vi "Coordinate_Outlier_Filtering_R1.vi"(0 "Num of Beacons":i8=5, 1 "Max Std Dev(all 5)":dbl=1.0, 5 "X in":sgl[](array[numeric]), 7 "Valid Data\nSets in":bool[](array[boolean])=[TRUE, TRUE, TRUE, TRUE, TRUE], 9 "Y in":sgl[](array[numeric]), 11 "Max Std Dev( 4 )":dbl=1.0, 13 "Max Std Dev (3)":dbl=1.0) -> (3 "Y out":sgl[](array[numeric]), 4 "Max":i32, 6 "Min Std Dev\nfor Max beacons":dbl, 8 "X out":sgl[](array[numeric]), 10 "Valid Beacons\nout":bool[](array[boolean]), 15 "Slope out":dbl)   [LabVIEW 2015]
uses:
  <vilib>/Analysis/NI_AALPro.lvlib
panel:
  out "std dev_current":dbl format="%0.6f"
  out "std dev_current 3":dbl format="%0.6f"
  out "size(s) 2":i32
  out "std dev_current 2":dbl format="%0.6f"
  out "size(s)":i32
  in  "Combo_info\nTemplate":T1={"Num Beacons"=0, "Std Dev_combo"=0.0, "Valid Data\nSets_combo"=[FALSE, FALSE, FALSE, FALSE, FALSE], "Slope combo"=0.0}
types:
  T1 = cluster{"Num Beacons":u8, "Std Dev_combo":dbl, "Valid Data\nSets_combo":bool[], "Slope combo":dbl}
  T2 = cluster{"dimension size":u8, sgl, bool[], "slope":dbl}
  T3 = cluster{"dimension size":u8, "Std Dev_combo":dbl, "Valid Data\nSets_combo":bool[], "slope":dbl}[]
  T4 = cluster{"dimension size":u8, dbl, bool[], "slope":dbl}
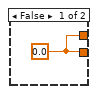
[diagram p2: hidden frame]
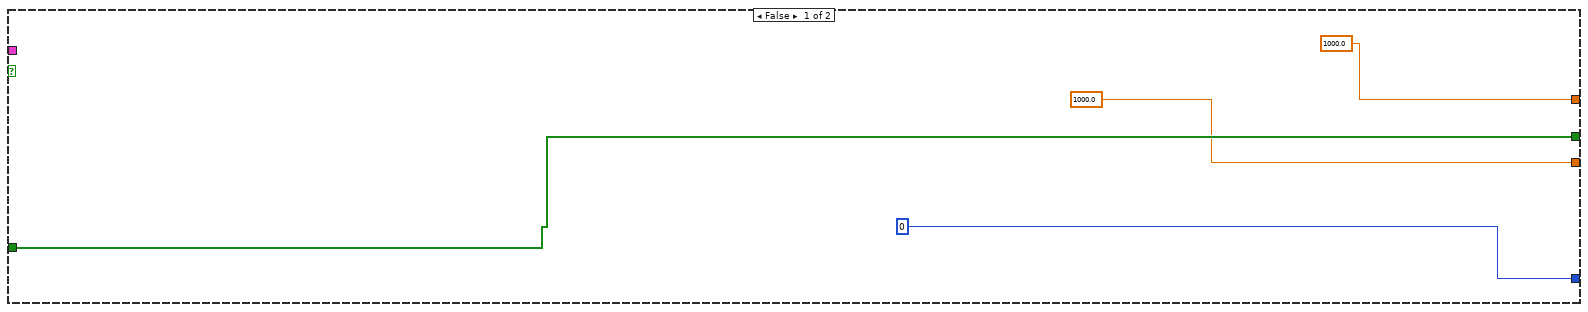
[diagram p3: hidden frame]
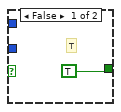
[diagram p8: hidden frame]
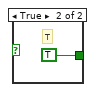
[diagram p9: hidden frame]
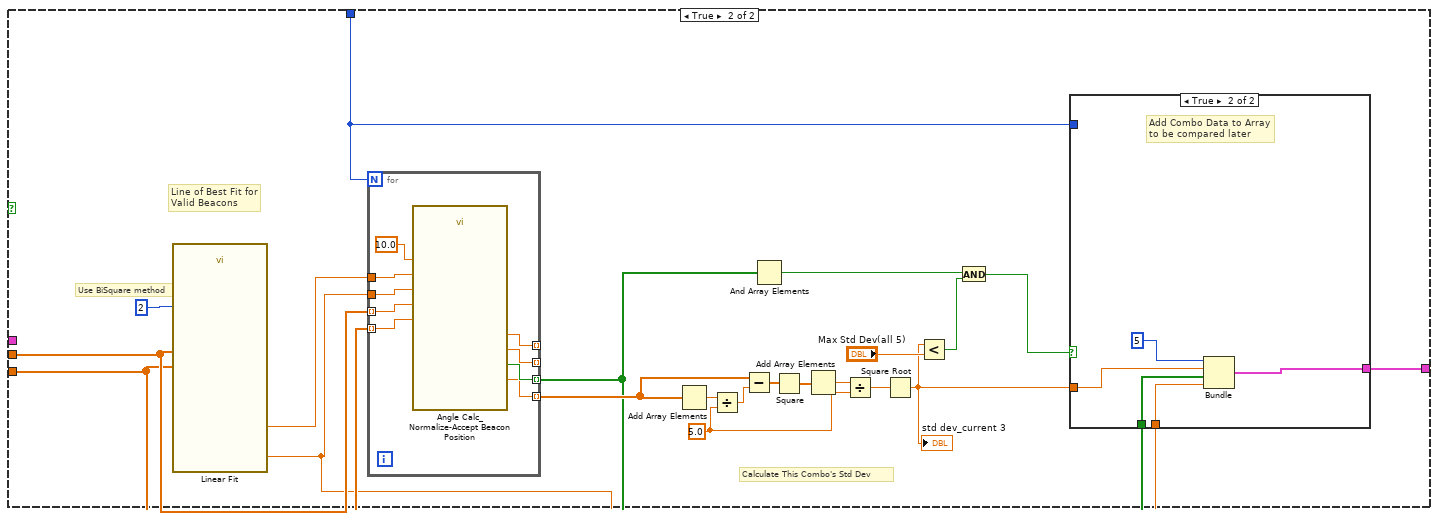
[diagram p13: hidden frame]
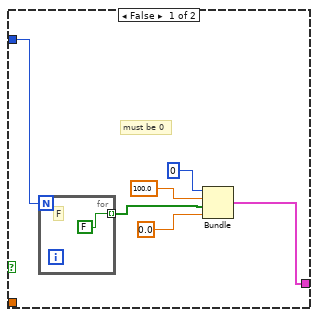
[diagram p14: hidden frame]
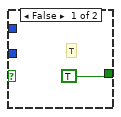
[diagram p16: hidden frame]
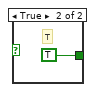
[diagram p17: hidden frame]
diagram:
  # "Use BiSquare method"
  # "Line of Best Fit for\nValid Beacons"
  # "5  Beacon Combination (only 1)"
  # "4 Beacon Combinations"
  # "3 Beacon Combinations"
  n1 = Boolean To (0,1)(Boolean="Valid Data\nSets in") -> (0, 1=w39:i16[])
  n2 = Add Array Elements(numeric array=w39) -> (sum=w26:i16)
  n3 = Equal?(x=w26, y=5 ("dimension size")) -> (x = y?=w34:bool)
  n4 = case shown="False" w34 {
    tunnel: "X in" -> [_ w59]
    tunnel: "Y in" -> [_ w58]
    tunnel: "Num of Beacons" -> [_ w43]
    tunnel: [w40 w44] -> w32
    tunnel: "Combo_info\nTemplate" -> [w40 _]
    frame False {
    }
    frame True {
      w42 = sgl 5.0 ("y")
      # "Calculate This Combo's Std Dev"
      # "Use BiSquare method"
      # "Line of Best Fit for\nValid Beacons"
      n5 = call <vilib>:"Linear Fit.vi"("Y"=w58, "X"=w59, "method"=2) -> ("slope"=w41:dbl, "intercept"=w60:dbl)  [unwired: 8 in, 3 out]
      n6 = for {
        N: w43 -> [_]
        tunnel: w41 -> [w81]
        tunnel: w60 -> [w80]
        tunnel: w59 -> [w79] mode=indexing
        tunnel: w58 -> [w78] mode=indexing
        tunnel: [w77] -> w45 mode=indexing
        tunnel: [w76] -> w46 mode=indexing
        tunnel: [w75] -> _ mode=indexing
        tunnel: [w74] -> _ mode=indexing
        n7 = call "Angle Calc_Normalize-Accept Beacon Position.vi"("slope"=w81, "Xin"=w79, "Deviation Threshold"=sgl 10.0 ("Deviation Threshold\n- Local Beacon Pos(*unit)"), "intercept"=w80, "Yin"=w78) -> ("Accept Beacon"=w77:bool, "Xout"=w75:sgl, "Distance"=w76:sgl, "Yout"=w74:sgl)  [unwired: 6 in, 1 out]
      }
      n8 = Add Array Elements(numeric array=w46) -> (sum=w57:sgl)
      n9 = Divide(x=w57, y=w42) -> (x/y=w56:sgl)
      n10 = Subtract(x=w46, y=w56) -> (x-y=w55:sgl[])
      n11 = And Array Elements(Boolean array=w45) -> (logical AND=w51:bool)
      n12 = Square(x=w55) -> (x^2=w47:sgl[])
      n13 = Add Array Elements(numeric array=w47) -> (sum=w53:sgl)
      n14 = Divide(x=w53, y=w42) -> (x/y=w54:sgl)
      n15 = Square Root(x=w54) -> (sqrt(x)=w49:sgl)
      "std dev_current 3" <- w49
      n16 = Less?(x=w49, y="Max Std Dev(all 5)") -> (x < y?=w50:bool)
      n17 = And(x=w51, y=w50) -> (x .and. y?=w48:bool)
      n18 = case shown="True" w48 {
        tunnel: w49 -> [_ w72]
        tunnel: w45 -> [_ w71]
        tunnel: [w64 w70] -> w44
        tunnel: w43 -> [w63 _]
        tunnel: w41 -> [_ w69]
        frame False {
          # "must be 0"
          n19 = for {
            N: w63 -> [_]
            tunnel: [FALSE] -> w65 mode=indexing
            # "F"
          }
          n20 = Bundle("dimension size"=u8 0, 100.0, w65, 0.0) -> (w64:cluster{"dimension size":u8, dbl, bool[], dbl})  [unwired: 1 in]
        }
        frame True {
          # "Add Combo Data to Array\nto be compared later"
          n21 = Bundle("dimension size"=u8 5, w72, w71, "slope"=w69) -> (w70:T2)  [unwired: 1 in]
        }
      }
    }
  }
  n22 = Build Array(w32) -> (w30:T3)
  n23 = Greater Or Equal?(x=w26, y=i16 4) -> (x >= y?=w37:bool)
  n24 = case shown="True" w37 {
    tunnel: "Num of Beacons" -> [_ w87]
    tunnel: "X in" -> [_ w90]
    tunnel: "Y in" -> [_ w89]
    tunnel: "Valid Data\nSets in" -> [_ w88]
    tunnel: w30 -> [w83 w86]
    tunnel: [w83 w85] -> w29
    tunnel: "Num of Beacons" -> [_ w84]
    frame False {
    }
    frame True {
      n25 = for {
        N: w87 -> [w94]
        shift-right: [w92] -> w85
        shift-left: w86 -> [w93]
        tunnel: w90 -> [w97]
        tunnel: w89 -> [w96]
        tunnel: w88 -> [w98]
        tunnel: w84 -> [w91]
        i -> [w95]
        n26 = for {
          N: w94 -> [w102]
          tunnel: w95 -> [w104]
          shift-right: [w100] -> w92
          shift-left: w93 -> [w101]
          tunnel: w97 -> [w106]
          tunnel: w96 -> [w105]
          tunnel: w98 -> [w107]
          tunnel: w91 -> [w99]
          i -> [w103]
          n27 = for {
            N: w102 -> [w110]
            tunnel: w107 -> [w116]
            tunnel: w106 -> [w115]
            tunnel: w105 -> [w114]
            tunnel: w104 -> [w111]
            tunnel: w103 -> [w117]
            shift-right: [w113] -> w100
            shift-left: w101 -> [w109]
            tunnel: w99 -> [w108]
            i -> [w112]
            n28 = for {
              N: w110 -> [w127]
              tunnel: w117 -> [w129]
              tunnel: w116 -> [w152]
              tunnel: w115 -> [w150]
              tunnel: w114 -> [w149]
              tunnel: w112 -> [w130]
              tunnel: w111 -> [w128]
              shift-right: [w139] -> w113
              shift-left: w109 -> [w131]
              tunnel: w108 -> [w118]
              i -> [w126]
              w132 = 4
              # "Build Beacon Set Boolean Array\n(correlates to indexes)"
              # "Fetch Coordinates"
              # "Are All Indexes Different?\nAND\nDo those indexes contain valid beacons?\nAND\nIs it not a repeat combo?"
              n29 = Greater?(x=w130, y=w129) -> (0:w122:bool)
              n30 = Greater?(x=w129, y=w128) -> (0:w123:bool)
              n31 = Greater?(x=w126, y=w130) -> (0:w121:bool)
              n32 = Build Array(w128, w129, w130, w126) -> (w137:i32[])
              n33 = for {
                N: w132 -> [_]
                tunnel: w137 -> [w156] mode=indexing
                tunnel: w137 -> [w157]
                tunnel: [w154] -> w136 mode=indexing
                tunnel: w132 -> [w153]
                i -> [w158]
                n34 = for {
                  N: w153 -> [_]
                  tunnel: w158 -> [w163]
                  tunnel: w157 -> [w161] mode=indexing
                  tunnel: w156 -> [w160]
                  tunnel: [w159] -> w155 mode=indexing
                  i -> [w162]
                  n35 = Not Equal?(x=w163, y=w162) -> (x != y?=w164:bool)
                  n36 = case shown="True" w164 {
                    tunnel: w161 -> [_ w167]
                    tunnel: w160 -> [_ w166]
                    tunnel: [TRUE w168] -> w159
                    frame False {
                      # "T"
                    }
                    frame True {
                      n37 = Not Equal?(x=w166, y=w167) -> (x != y?=w168:bool)
                    }
                  }
                }
                n38 = And Array Elements(Boolean array=w155) -> (logical AND=w154:bool)
              }
              n39 = And Array Elements(Boolean array=w136) -> (logical AND=w120:bool)
              n40 = Index Array(array=w150, index #1=w128, index #2=w129, index #3=w130, index #4=w126) -> (element #1=w148:sgl, element #2=w147:sgl, element #3=w146:sgl, element #4=w125:sgl)
              n41 = Index Array(array=w149, index #1=w128, index #2=w129, index #3=w130, index #4=w126) -> (element #1=w145:sgl, element #2=w144:sgl, element #3=w143:sgl, element #4=w124:sgl)
              n42 = Index Array(array=w152, index #1=w128, index #2=w129, index #3=w130, index #4=w126) -> (element #1=w135:bool, element #2=w134:bool, element #3=w133:bool, element #4=w119:bool)
              n43 = for {
                N: w127 -> [_]
                tunnel: w130 -> [w179]
                tunnel: w129 -> [w178]
                tunnel: w128 -> [w177]
                tunnel: [w172] -> w138 mode=indexing
                tunnel: w126 -> [w170]
                i -> [w171]
                n44 = Equal?(x=w177, y=w171) -> (x = y?=w174:bool)
                n45 = Equal?(x=w179, y=w171) -> (x = y?=w176:bool)
                n46 = Equal?(x=w178, y=w171) -> (x = y?=w175:bool)
                n47 = Equal?(x=w170, y=w171) -> (x = y?=w169:bool)
                n48 = Compound Arithmetic op=OR(w176, w175, w174, w169) -> (w173:bool)
                n49 = case shown="False" w173 {
                  tunnel: [FALSE TRUE] -> w172
                  frame False {
                    # "F"
                  }
                  frame True {
                    # "T"
                  }
                }
              }
              n50 = Build Array(w148, w147, w146, w125) -> (w142:sgl[])
              n51 = Build Array(w145, w144, w143, w124) -> (w141:sgl[])
              n52 = Build Array(w135, w134, w133, w119) -> (w140:bool[])
              n53 = Compound Arithmetic op=AND(w135, w134, w133, w119, w120, w121, w122, w123) -> (w151:bool)
              n54 = case shown="True" w151 {
                tunnel: w142 -> [_ w200]
                tunnel: w141 -> [_ w201]
                tunnel: w140 -> [_ w191]
                tunnel: w131 -> [w182 w189]
                tunnel: [w182 w187] -> w139
                tunnel: w138 -> [_ w185]
                tunnel: w118 -> [_ w184]
                frame False {
                }
                frame True {
                  # "Calculate Distance from\nBeacon to Fitted Line"
                  # "Calculate This Combo's Std Dev"
                  # "Trim Arrays to Only Valid Beacons"
                  # "Use BiSquare method"
                  # "Line of Best Fit for\nValid Beacons"
                  # "All Indexes are Different and Beacons are Valid"
                  n55 = Initialize Array(sgl 0.0 ("element"), 4 ("dimension size")) -> (w209:sgl[])
                  n56 = for {
                    N: w184 -> [_]
                    shift-right: [w228] -> w198
                    shift-left: 0.0 -> [w229]
                    shift-right: [w227] -> w203
                    shift-left: w209 -> [w226]
                    shift-right: [w224] -> w202
                    shift-left: w209 -> [w225]
                    tunnel: w191 -> [w223] mode=indexing
                    tunnel: w200 -> [w222] mode=indexing
                    tunnel: w201 -> [w221] mode=indexing
                    n57 = case shown="True" w223 {
                      tunnel: w229 -> [w232 w239]
                      tunnel: [w232 w240] -> w228
                      tunnel: [w231 w237] -> w227
                      tunnel: w226 -> [w231 w236]
                      tunnel: w225 -> [w230 w235]
                      tunnel: [w230 w238] -> w224
                      tunnel: w222 -> [_ w234]
                      tunnel: w221 -> [_ w233]
                      frame False {
                      }
                      frame True {
                        n58 = Replace Array Subset(array=w236, new element=w234, index=w239) -> (w237:sgl[])
                        n59 = Replace Array Subset(array=w235, new element=w233, index=w239) -> (w238:sgl[])
                        n60 = Increment(x=w239) -> (x+1=w240:dbl)
                      }
                    }
                  }
                  n61 = call <vilib>:"Linear Fit.vi"("Y"=w202, "X"=w203, "method"=2) -> ("slope"=w183:dbl, "intercept"=w211:dbl)  [unwired: 8 in, 3 out]
                  n62 = for {
                    N: w184 -> [_]
                    tunnel: w211 -> [w249]
                    tunnel: w183 -> [w248]
                    tunnel: w203 -> [w247] mode=indexing
                    tunnel: w202 -> [w246] mode=indexing
                    tunnel: [w245] -> w194 mode=indexing
                    tunnel: [w244] -> _ mode=indexing
                    tunnel: [w243] -> _ mode=indexing
                    tunnel: [w242] -> w196 mode=indexing
                    n63 = call "Angle Calc_Normalize-Accept Beacon Position.vi"("slope"=w248, "Xin"=w247, "Deviation Threshold"=sgl 10.0 ("Deviation Threshold\n- Local Beacon Pos(*unit)"), "intercept"=w249, "Yin"=w246) -> ("Accept Beacon"=w245:bool, "Xout"=w244:sgl, "Distance"=w242:sgl, "Yout"=w243:sgl)  [unwired: 6 in, 1 out]
                  }
                  n64 = Add Array Elements(numeric array=w196) -> (sum=w208:sgl)
                  n65 = Divide(x=w208, y=w198) -> (x/y=w207:dbl)
                  n66 = Subtract(x=w196, y=w207) -> (x-y=w206:dbl[])
                  n67 = And Array Elements(Boolean array=w194) -> (logical AND=w193:bool)
                  n68 = Square(x=w206) -> (x^2=w195:dbl[])
                  n69 = Add Array Elements(numeric array=w195) -> (sum=w204:dbl)
                  n70 = Divide(x=w204, y=w198) -> (x/y=w205:dbl)
                  n71 = Square Root(x=w205) -> (sqrt(x)=w190:dbl)
                  "std dev_current 2" <- w190
                  n72 = Less?(x=w190, y="Max Std Dev( 4 )") -> (x < y?=w192:bool)
                  n73 = And(x=w193, y=w192) -> (x .and. y?=w188:bool)
                  n74 = case shown="True" w188 {
                    tunnel: w185 -> [_ w220]
                    tunnel: w190 -> [_ w219]
                    tunnel: w189 -> [w213 w218]
                    tunnel: [w213 w217] -> w187
                    tunnel: w183 -> [_ w214]
                    frame False {
                    }
                    frame True {
                      # "Add Combo Data to Array\nto be compared later"
                      n75 = Bundle("dimension size"=u8 4, w219, w220, "slope"=w214) -> (w215:T4)  [unwired: 1 in]
                      n76 = Build Array (concatenate)(w218, w215) -> (w217:T3)
                    }
                  }
                }
              }
            }
          }
        }
      }
    }
  }
  n77 = Array Size(array=w29) -> (size(s)=w35:i32)
  n78 = Decrement(x=w35) -> (x-1=w24:i32)
  "size(s) 2" <- w24
  n79 = Greater Or Equal?(x=w26, y=3 ("dimension size")) -> (x >= y?=w27:bool)
  n80 = case shown="True" w27 {
    tunnel: "Num of Beacons" -> [_ w251]
    tunnel: "X in" -> [_ w256]
    tunnel: "Y in" -> [_ w255]
    tunnel: "Valid Data\nSets in" -> [_ w254]
    tunnel: w29 -> [w250 w253]
    tunnel: [w250 w252] -> w21
    frame False {
    }
    frame True {
      n81 = for {
        N: w251 -> [w259]
        shift-right: [w257] -> w252
        shift-left: w253 -> [w258]
        tunnel: w256 -> [w262]
        tunnel: w255 -> [w261]
        tunnel: w254 -> [w263]
        i -> [w260]
        n82 = for {
          N: w259 -> [w266]
          tunnel: w260 -> [w268]
          shift-right: [w264] -> w257
          shift-left: w258 -> [w265]
          tunnel: w262 -> [w270]
          tunnel: w261 -> [w269]
          tunnel: w263 -> [w271]
          i -> [w267]
          n83 = for {
            N: w266 -> [w282]
            tunnel: w271 -> [w300]
            tunnel: w270 -> [w298]
            tunnel: w269 -> [w297]
            tunnel: w268 -> [w272]
            tunnel: w267 -> [w273]
            shift-right: [w283] -> w264
            shift-left: w265 -> [w284]
            i -> [w274]
            w279 = 3
            # "Build Beacon Set Boolean Array\n(correlates to indexes)"
            # "Fetch Coordinates"
            # "Are All Indexes Different?\nAND\nDo those indexes contain valid beacons?\nAND\nIs it not a repeat combo?"
            n84 = Greater?(x=w274, y=w273) -> (0:w276:bool)
            n85 = Greater?(x=w273, y=w272) -> (0:w275:bool)
            n86 = Build Array(w272, w273, w274) -> (w280:i32[])
            n87 = for {
              N: w279 -> [_]
              tunnel: w280 -> [w304] mode=indexing
              tunnel: w280 -> [w305]
              tunnel: [w302] -> w278 mode=indexing
              tunnel: w279 -> [w301]
              i -> [w306]
              n88 = for {
                N: w301 -> [_]
                tunnel: w306 -> [w311]
                tunnel: w305 -> [w309] mode=indexing
                tunnel: w304 -> [w308]
                tunnel: [w307] -> w303 mode=indexing
                i -> [w310]
                n89 = Not Equal?(x=w311, y=w310) -> (x != y?=w312:bool)
                n90 = case shown="True" w312 {
                  tunnel: w309 -> [_ w315]
                  tunnel: w308 -> [_ w314]
                  tunnel: [TRUE w316] -> w307
                  frame False {
                    # "T"
                  }
                  frame True {
                    n91 = Not Equal?(x=w314, y=w315) -> (x != y?=w316:bool)
                  }
                }
              }
              n92 = And Array Elements(Boolean array=w303) -> (logical AND=w302:bool)
            }
            n93 = And Array Elements(Boolean array=w278) -> (logical AND=w277:bool)
            n94 = Index Array(array=w298, index #1=w272, index #2=w273, index #3=w274) -> (element #1=w296:sgl, element #2=w295:sgl, element #3=w294:sgl)
            n95 = Index Array(array=w297, index #1=w272, index #2=w273, index #3=w274) -> (element #1=w293:sgl, element #2=w292:sgl, element #3=w291:sgl)
            n96 = for {
              N: w282 -> [_]
              tunnel: w274 -> [w324]
              tunnel: w273 -> [w323]
              tunnel: w272 -> [w322]
              tunnel: [w317] -> w281 mode=indexing
              i -> [w325]
              n97 = Equal?(x=w322, y=w325) -> (x = y?=w319:bool)
              n98 = Equal?(x=w324, y=w325) -> (x = y?=w321:bool)
              n99 = Equal?(x=w323, y=w325) -> (x = y?=w320:bool)
              n100 = Compound Arithmetic op=OR(w321, w320, w319) -> (w318:bool)
              n101 = case shown="False" w318 {
                tunnel: [FALSE TRUE] -> w317
                frame False {
                  # "F"
                }
                frame True {
                  # "T"
                }
              }
            }
            n102 = Index Array(array=w300, index #1=w272, index #2=w273, index #3=w274) -> (element #1=w288:bool, element #2=w290:bool, element #3=w289:bool)
            n103 = Build Array(w296, w295, w294) -> (w287:sgl[])
            n104 = Build Array(w293, w292, w291) -> (w286:sgl[])
            n105 = Build Array(w288, w290, w289) -> (w285:bool[])
            n106 = Compound Arithmetic op=AND(w288, w290, w289, w277, w276, w275) -> (w299:bool)
            n107 = case shown="True" w299 {
              tunnel: w287 -> [_ w346]
              tunnel: w286 -> [_ w347]
              tunnel: w285 -> [_ w337]
              tunnel: w282 -> [_ w332]
              tunnel: w284 -> [w328 w335]
              tunnel: [w328 w333] -> w283
              tunnel: w281 -> [_ w330]
              frame False {
              }
              frame True {
                # "Calculate Distance from\nBeacon to Fitted Line"
                # "Calculate This Combo's Std Dev"
                # "Trim Arrays to Only Valid Beacons"
                # "Use BiSquare method"
                # "Line of Best Fit for\nValid Beacons"
                # "All Indexes are Different and Beacons are Valid"
                n108 = Initialize Array(sgl 0.0 ("element"), 3 ("dimension size")) -> (w355:sgl[])
                n109 = for {
                  N: w332 -> [_]
                  shift-right: [w374] -> w344
                  shift-left: 0.0 -> [w375]
                  shift-right: [w373] -> w349
                  shift-left: w355 -> [w372]
                  shift-right: [w370] -> w348
                  shift-left: w355 -> [w371]
                  tunnel: w337 -> [w369] mode=indexing
                  tunnel: w346 -> [w368] mode=indexing
                  tunnel: w347 -> [w367] mode=indexing
                  n110 = case shown="True" w369 {
                    tunnel: w375 -> [w378 w385]
                    tunnel: [w378 w386] -> w374
                    tunnel: [w377 w383] -> w373
                    tunnel: w372 -> [w377 w382]
                    tunnel: w371 -> [w376 w381]
                    tunnel: [w376 w384] -> w370
                    tunnel: w368 -> [_ w380]
                    tunnel: w367 -> [_ w379]
                    frame False {
                    }
                    frame True {
                      n111 = Replace Array Subset(array=w382, new element=w380, index=w385) -> (w383:sgl[])
                      n112 = Replace Array Subset(array=w381, new element=w379, index=w385) -> (w384:sgl[])
                      n113 = Increment(x=w385) -> (x+1=w386:dbl)
                    }
                  }
                }
                n114 = call <vilib>:"Linear Fit.vi"("Y"=w348, "X"=w349, "method"=2) -> ("slope"=w329:dbl, "intercept"=w357:dbl)  [unwired: 8 in, 3 out]
                n115 = for {
                  N: w332 -> [_]
                  tunnel: w357 -> [w395]
                  tunnel: w329 -> [w394]
                  tunnel: w349 -> [w393] mode=indexing
                  tunnel: w348 -> [w392] mode=indexing
                  tunnel: [w391] -> w340 mode=indexing
                  tunnel: [w390] -> _ mode=indexing
                  tunnel: [w389] -> _ mode=indexing
                  tunnel: [w388] -> w342 mode=indexing
                  n116 = call "Angle Calc_Normalize-Accept Beacon Position.vi"("slope"=w394, "Xin"=w393, "Deviation Threshold"=sgl 10.0 ("Deviation Threshold\n- Local Beacon Pos(*unit)"), "intercept"=w395, "Yin"=w392) -> ("Accept Beacon"=w391:bool, "Xout"=w390:sgl, "Distance"=w388:sgl, "Yout"=w389:sgl)  [unwired: 6 in, 1 out]
                }
                n117 = Add Array Elements(numeric array=w342) -> (sum=w354:sgl)
                n118 = Divide(x=w354, y=w344) -> (x/y=w353:dbl)
                n119 = Subtract(x=w342, y=w353) -> (x-y=w352:dbl[])
                n120 = And Array Elements(Boolean array=w340) -> (logical AND=w339:bool)
                n121 = Square(x=w352) -> (x^2=w341:dbl[])
                n122 = Add Array Elements(numeric array=w341) -> (sum=w350:dbl)
                n123 = Divide(x=w350, y=w344) -> (x/y=w351:dbl)
                n124 = Square Root(x=w351) -> (sqrt(x)=w336:dbl)
                "std dev_current" <- w336
                n125 = Less?(x=w336, y="Max Std Dev (3)") -> (x < y?=w338:bool)
                n126 = And(x=w339, y=w338) -> (x .and. y?=w334:bool)
                n127 = case shown="True" w334 {
                  tunnel: w330 -> [_ w366]
                  tunnel: w336 -> [_ w365]
                  tunnel: w335 -> [w359 w364]
                  tunnel: [w359 w363] -> w333
                  tunnel: w329 -> [_ w360]
                  frame False {
                  }
                  frame True {
                    # "Add Combo Data to Array\nto be compared later"
                    n128 = Bundle("dimension size"=u8 3, w365, w366, "slope"=w360) -> (w361:T4)  [unwired: 1 in]
                    n129 = Build Array (concatenate)(w364, w361) -> (w363:T3)
                  }
                }
              }
            }
          }
        }
      }
    }
  }
  n130 = Array Size(array=w21) -> (size(s)=w2:i32)
  n131 = Initialize Array(FALSE, 5 ("dimension size")) -> (w15:bool[])
  n132 = Greater Than 0?(x=w2) -> (x > 0?=w20:bool)
  n133 = case shown="True" w20 {
    tunnel: w2 -> [_ w407]
    tunnel: w21 -> [_ w409]
    tunnel: [1000.0 w406] -> w19
    tunnel: [0 w405] -> w18
    tunnel: [w398 w404] -> w3
    tunnel: w15 -> [w398 w403]
    tunnel: [1000.0 w402] -> w14
    frame False {
    }
    frame True {
      # "Pick Lowest Std Deviation\nfrom Combos with Max"
      # "Max"
      # "Find Combo with\nMax Number of Beacons"
      n134 = for {
        N: w407 -> [_]
        tunnel: w409 -> [w448] mode=indexing
        shift-right: [w446] -> w405
        shift-left: 0 -> [w444]
        n135 = Unbundle(w448) -> ("dimension size"=w445:u8)  [unwired: 3 out]
        n136 = Greater?(x=w445, y=w444) -> (0:w447:bool)
        n137 = case shown="True" w447 {
          tunnel: [w449 w450] -> w446
          tunnel: w445 -> [_ w450]
          tunnel: w444 -> [w449 _]
          frame False {
          }
          frame True {
            # "New Max"
          }
        }
      }
      n138 = Greater Than 0?(x=w405) -> (x > 0?=w408:bool)
      n139 = case shown="True" w408 {
        tunnel: w405 -> [_ w422]
        tunnel: w409 -> [_ w421]
        tunnel: w407 -> [_ w420]
        tunnel: [w412 w419] -> w406
        tunnel: [w413 w418] -> w404
        tunnel: w403 -> [w413 w417]
        tunnel: [w411 w416] -> w402
        tunnel: 1000.0 -> [w411 w415]
        tunnel: 1000.0 -> [w412 w414]
        frame False {
        }
        frame True {
          # "Min\nStd Dev"
          n140 = for {
            N: w420 -> [_]
            shift-right: [w437] -> w419
            shift-left: w414 -> [w436]
            tunnel: w421 -> [w435] mode=indexing
            tunnel: w422 -> [w434]
            shift-right: [w428] -> w418
            shift-left: w417 -> [w426]
            shift-right: [w424] -> w416
            shift-left: w415 -> [w423]
            n141 = Unbundle(w435) -> ("dimension size"=w433:u8, "Std Dev_combo"=w429:dbl, "Valid Data\nSets_combo"=w427:bool[], "slope"=w425:dbl)
            n142 = Less?(x=w429, y=w436) -> (x < y?=w430:bool)
            n143 = Equal?(x=w434, y=w433) -> (x = y?=w431:bool)
            n144 = And(x=w431, y=w430) -> (x .and. y?=w432:bool)
            n145 = case shown="True" w432 {
              tunnel: [w440 w443] -> w437
              tunnel: w436 -> [w440 _]
              tunnel: w429 -> [_ w443]
              tunnel: [w439 w442] -> w428
              tunnel: w427 -> [_ w442]
              tunnel: w426 -> [w439 _]
              tunnel: [w438 w441] -> w424
              tunnel: w425 -> [_ w441]
              tunnel: w423 -> [w438 _]
              frame False {
              }
              frame True {
                # "New Max"
              }
            }
          }
        }
      }
    }
  }
  "Min Std Dev\nfor Max beacons" <- w19
  "Max" <- w18
  "Valid Beacons\nout" <- w3
  "Slope out" <- w14
  n146 = Array Size(array=w21) -> (size(s)=w38:i32)
  n147 = Decrement(x=w38) -> (x-1=w23:i32)
  n148 = Subtract(x=w23, y=w24) -> (x-y=→"size(s)":i32)
  n149 = Boolean To (0,1)(Boolean=w3) -> (0, 1=w10:i16[])
  n150 = Add(x=w10, y=1e-12) -> (x+y=w8:dbl[])
  n151 = call <vilib>:"Linear Fit.vi"("Y"="Y in", "X"="X in", "Weight"=w8, "method"=2) -> ("slope"=w11:dbl, "intercept"=w12:dbl)  [unwired: 7 in, 3 out]
  n152 = for {
    N: "Num of Beacons" -> [_]
    tunnel: w11 -> [w457]
    tunnel: w12 -> [w456]
    tunnel: "X in" -> [w455] mode=indexing
    tunnel: "Y in" -> [w454] mode=indexing
    tunnel: [w453] -> w5 mode=indexing
    tunnel: [w452] -> w4 mode=indexing
    tunnel: w3 -> [w451] mode=indexing
    n153 = case shown="True" w451 {
      tunnel: sgl 10.0 ("Deviation Threshold\n- Local Beacon Pos(*unit)") -> [_ w466]
      tunnel: w457 -> [_ w465]
      tunnel: w456 -> [_ w464]
      tunnel: w455 -> [_ w463]
      tunnel: w454 -> [_ w462]
      tunnel: [w459 w461] -> w453
      tunnel: [w459 w460] -> w452
      frame False {
        w459 = sgl 0.0
      }
      frame True {
        n154 = call "Angle Calc_Normalize-Accept Beacon Position.vi"("slope"=w465, "Xin"=w463, "Deviation Threshold"=w466, "intercept"=w464, "Yin"=w462) -> ("Xout"=w461:sgl, "Yout"=w460:sgl)  [unwired: 6 in, 3 out]
      }
    }
  }
  "X out" <- w5
  "Y out" <- w4
